vi "Move Turret (TRIAX).vi"(7 "Mono System # (0)":T2, 8 "error in (no error)":errorcluster, 10 "turret position (0)":T1, 11 "VISA resource name":refnum<visa-resource-name>) -> (0 "error out":errorcluster, 3 "VISA resource name out":refnum<visa-resource-name>)   [LabVIEW 2023, in "JY-SPEX-TRIAX.lvlib"]
doc: "Moves the turret to position 0, 1, or 2.\n\n<B>Note: works with TRIAX series spectrometers only.</B>"
uses:
  JY-SPEX-TRIAX.lvlib
  controls.llb/Monochromator System Number.ctl
  controls.llb/Turret Position (TRIAX).ctl
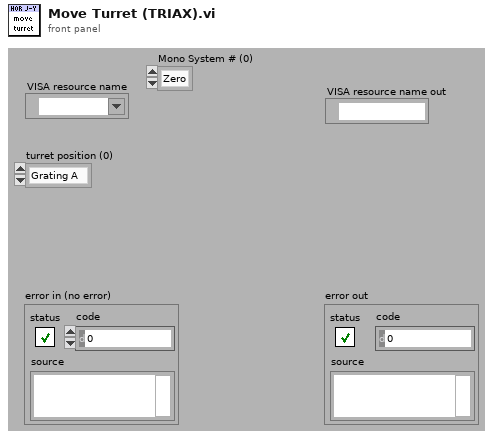
[diagram p1: front panel]
types:
  T1 = typedef "JY-SPEX-TRIAX.lvlib/Turret Position (TRIAX).ctl" = enum16{"Grating A", "Grating B", "Grating C"}
  T2 = typedef "JY-SPEX-TRIAX.lvlib/Monochromator System Number.ctl" = enum16{"Zero", "One"}
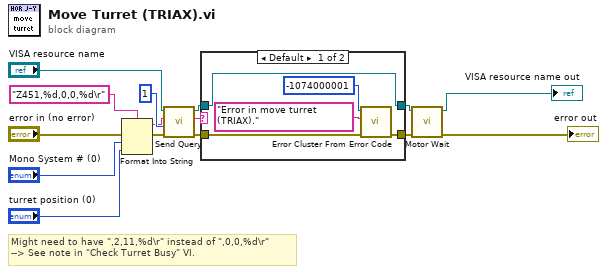
[diagram p0: block diagram]
diagram:
  # "Might need to have \",2,11,%d\\r\" instead of \",0,0,%d\\r\"\n--> See note in \"Check Turret Busy\" VI."
  n1 = Format Into String(format string="Z451,%d,0,0,%d\r", error in="error in (no error)", "Mono System # (0)", "turret position (0)") -> (resulting string=w7:string, error out=w5:errorcluster)  [unwired: 1 in]
  n2 = call "Send Query.vi"("error in (no error)"=w5, "byte count"=u32 1, "write buffer"=w7, "VISA resource name"="VISA resource name") -> ("error out"=w11:errorcluster, "read buffer"=w13:string, "VISA resource name out"=w12:refnum<visa-resource-name>)  [unwired: 5 out]
  n3 = case shown="Default" w13 {
    tunnel: w12 -> [w16 w22]
    tunnel: [w16 w22] -> w2
    tunnel: w11 -> [w18 w21]
    tunnel: [w17 w21] -> w4
    frame Default {
      n4 = call <vilib>:"Error Cluster From Error Code.vi"("error in (no error)"=w18, "error message (\"\")"="Error in move turret (TRIAX)." ("error message (\"\")"), "error code (0)"=-1074000001) -> ("error out"=w17:errorcluster)  [unwired: 1 in, 5 out]
    }
    frame "o" {
    }
  }
  n5 = call "Motor Wait.vi"("error in"=w4, "VISA resource name in"=w2) -> ("error out"=→"error out":errorcluster, "VISA resource name out"=→"VISA resource name out":refnum<visa-resource-name>)  [unwired: 8 out]
